vi "FomatDTCPN.vi"(8 "PN_Format":string, 9 "Manufacturer":string, 10 "SWVersion":string, 11 "Part Number (Palet Info)":string) -> (0 "Calculated PN Length":i32, 3 "Calc Part Number":string)   [LabVIEW 2017]
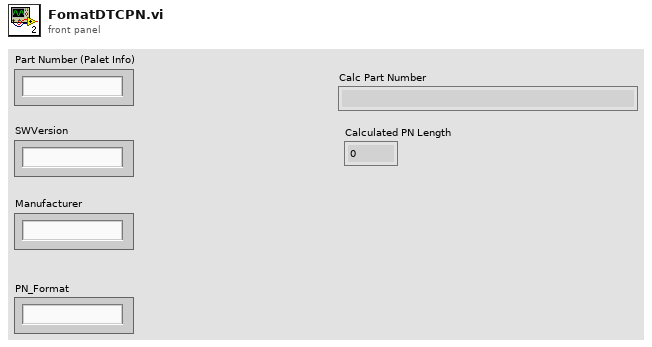
[diagram p1: front panel]
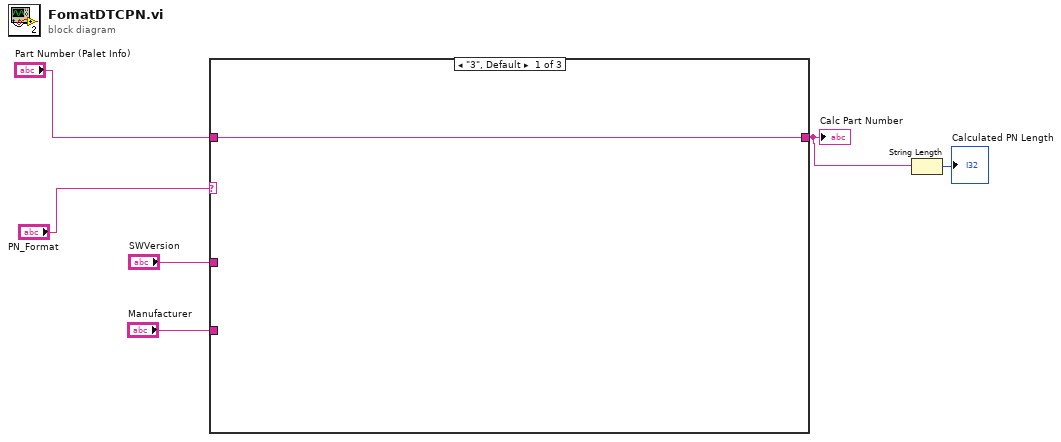
[diagram p0: block diagram]
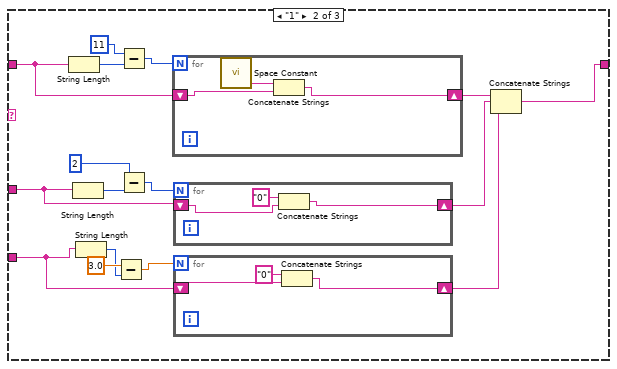
[diagram p2: hidden frame]
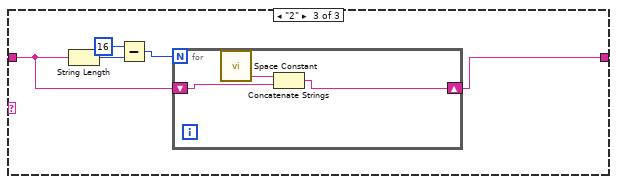
[diagram p3: hidden frame]
diagram:
  n1 = case shown="\"3\", Default" "PN_Format" {
    tunnel: "Part Number (Palet Info)" -> [w7 w21 w35]
    tunnel: [w7 w18 w33] -> w4
    tunnel: "SWVersion" -> [_ w14 _]
    tunnel: "Manufacturer" -> [_ w9 _]
    frame "3", Default {
    }
    frame "1" {
      n2 = String Length(string=w21) -> (length=w23:i32)
      n3 = String Length(string=w14) -> (length=w17:i32)
      n4 = String Length(string=w9) -> (length=w11:i32)
      n5 = Subtract(x=3.0, y=w11) -> (x-y=w10:dbl)
      n6 = Subtract(x=11, y=w23) -> (x-y=w20:i32)
      n7 = Subtract(x=2, y=w17) -> (x-y=w15:i32)
      n8 = for {
        N: w20 -> [_]
        shift-right: [w30] -> w19
        shift-left: w21 -> [w31]
        n9 = call <vilib>:"Space Constant.vi"() -> ("String"=w32:string)
        n10 = Concatenate Strings(w32, w31) -> (w30:string)
      }
      n11 = for {
        N: w15 -> [_]
        shift-right: [w27] -> w13
        shift-left: w14 -> [w28]
        n12 = Concatenate Strings("0" ("string"), w28) -> (w27:string)
      }
      n13 = for {
        N: w10 -> [_]
        shift-right: [w24] -> w8
        shift-left: w9 -> [w26]
        n14 = Concatenate Strings("0" ("string"), w26) -> (w24:string)
      }
      n15 = Concatenate Strings(w19, w13, w8) -> (w18:string)
    }
    frame "2" {
      n16 = String Length(string=w35) -> (length=w37:i32)
      n17 = Subtract(x=16, y=w37) -> (x-y=w34:i32)
      n18 = for {
        N: w34 -> [_]
        shift-right: [w38] -> w33
        shift-left: w35 -> [w39]
        n19 = call <vilib>:"Space Constant.vi"() -> ("String"=w40:string)
        n20 = Concatenate Strings(w40, w39) -> (w38:string)
      }
    }
  }
  "Calc Part Number" <- w4
  n21 = String Length(string=w4) -> (length=→"Calculated PN Length":i32)
